vi "MAVLink Driver Main.vi"(8 "error IO":errorcluster) -> ()   [LabVIEW 2014]
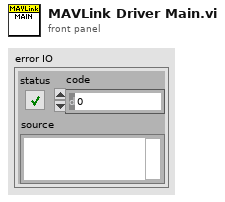
[diagram p1: front panel]
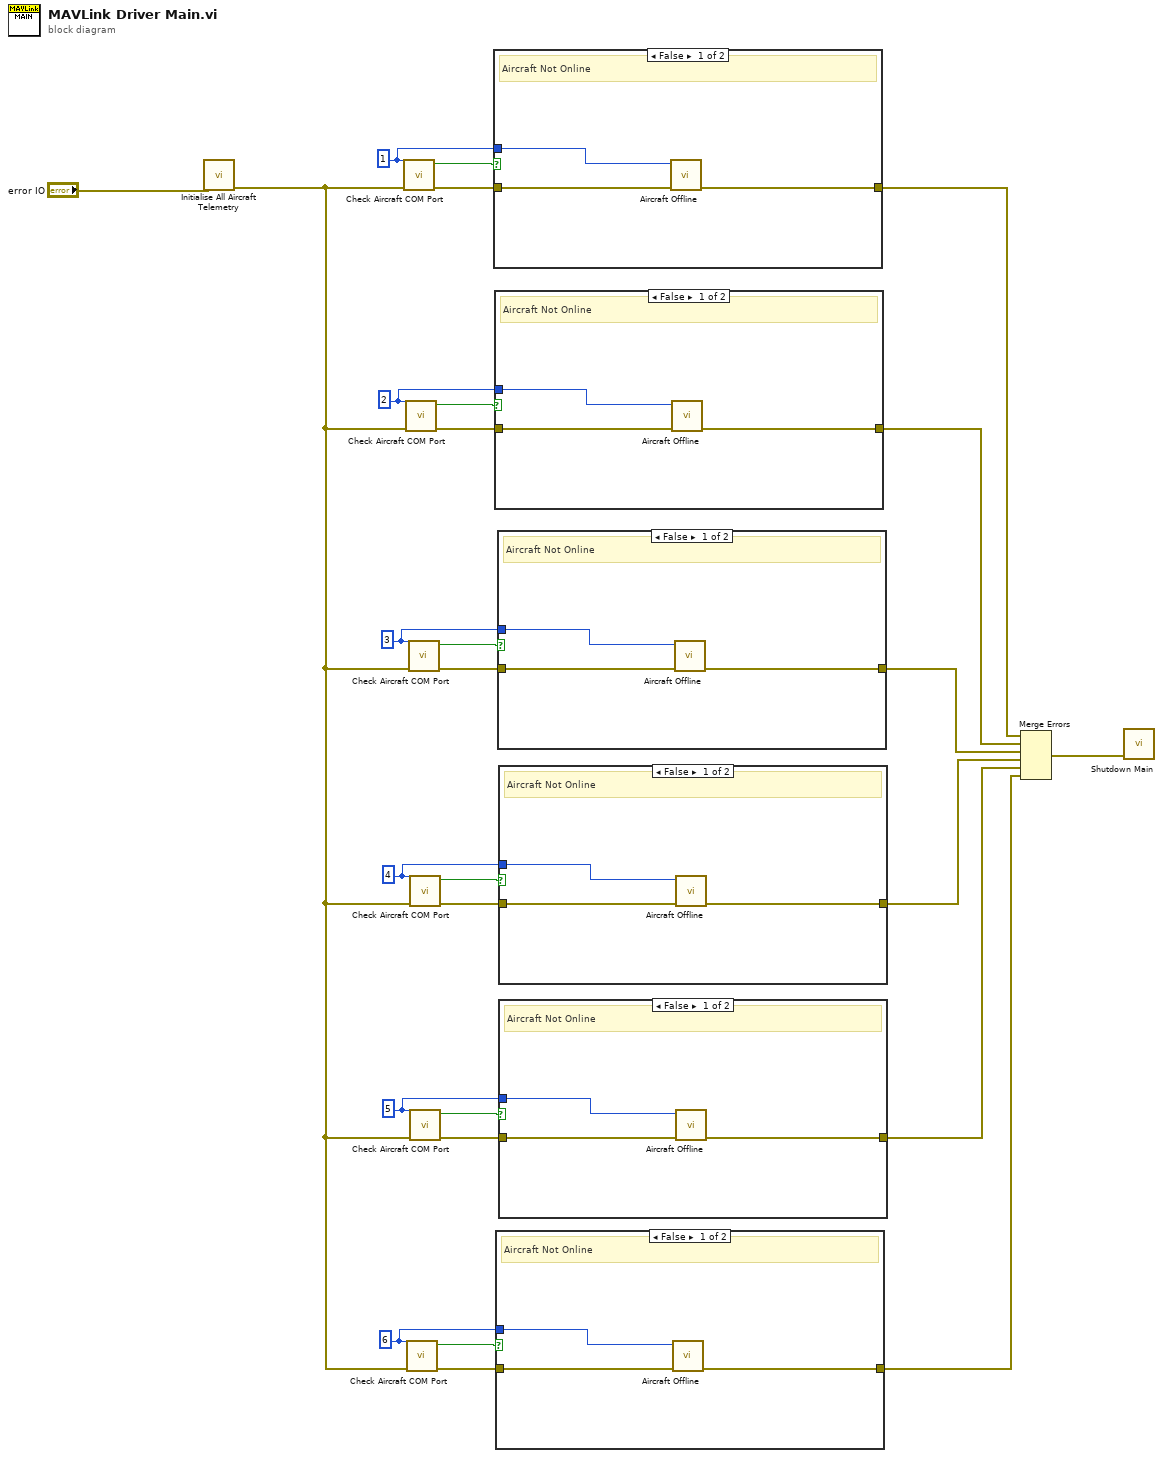
[diagram p0: block diagram]
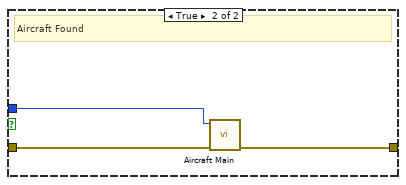
[diagram p2: hidden frame]
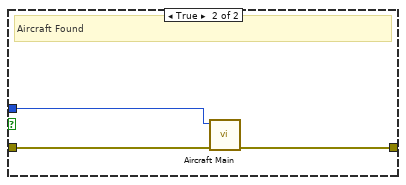
[diagram p3: hidden frame]
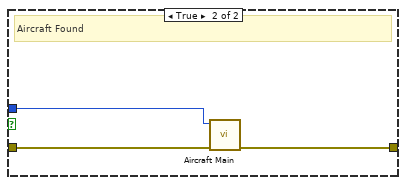
[diagram p4: hidden frame]
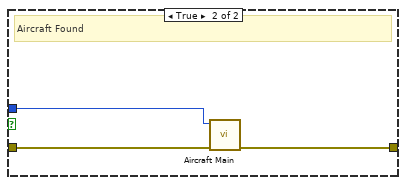
[diagram p5: hidden frame]
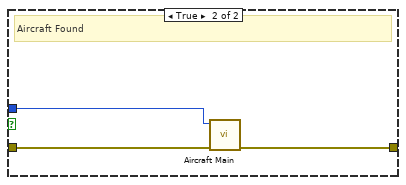
[diagram p6: hidden frame]
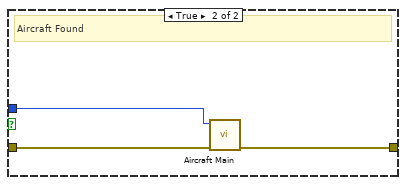
[diagram p7: hidden frame]
diagram:
  w11 = u8 6 ("Aircraft ID")
  w12 = u8 5 ("Aircraft ID")
  w17 = u8 4 ("Aircraft ID")
  w18 = u8 3 ("Aircraft ID")
  w23 = u8 2 ("Aircraft ID")
  w24 = u8 1 ("Aircraft ID")
  n1 = call "Initialise All Aircraft Telemetry.vi"("error IO"="error IO") -> ("error out"=w8:errorcluster)  [unwired: 10 in]
  n2 = call "Check Aircraft COM Port.vi"("Error In"=w8, "Aircraft ID"=w24) -> ("Error Out"=w25:errorcluster, "COM Port Found"=w26:bool)  [unwired: 8 in]
  n3 = call "Check Aircraft COM Port.vi"("Error In"=w8, "Aircraft ID"=w23) -> ("Error Out"=w22:errorcluster, "COM Port Found"=w21:bool)  [unwired: 8 in]
  n4 = call "Check Aircraft COM Port.vi"("Error In"=w8, "Aircraft ID"=w11) -> ("Error Out"=w10:errorcluster, "COM Port Found"=w9:bool)  [unwired: 8 in]
  n5 = call "Check Aircraft COM Port.vi"("Error In"=w8, "Aircraft ID"=w18) -> ("Error Out"=w19:errorcluster, "COM Port Found"=w20:bool)  [unwired: 8 in]
  n6 = call "Check Aircraft COM Port.vi"("Error In"=w8, "Aircraft ID"=w17) -> ("Error Out"=w16:errorcluster, "COM Port Found"=w15:bool)  [unwired: 8 in]
  n7 = call "Check Aircraft COM Port.vi"("Error In"=w8, "Aircraft ID"=w12) -> ("Error Out"=w13:errorcluster, "COM Port Found"=w14:bool)  [unwired: 8 in]
  n8 = case shown="False" w26 {
    tunnel: w25 -> [w29 w33]
    tunnel: w24 -> [w30 w32]
    tunnel: [w28 w31] -> w7
    frame False {
      # "Aircraft Not Online"
      n9 = call "Aircraft Offline.vi"("Error In"=w29, "Aircraft ID"=w30) -> ("Error Out"=w28:errorcluster)  [unwired: 9 in]
    }
    frame True {
      # "Aircraft Found"
      n10 = call "Aircraft Main.vi"("error out"=w33, "Aircraft Index"=w32) -> ("error out 2"=w31:errorcluster)  [unwired: 9 in]
    }
  }
  n11 = case shown="False" w21 {
    tunnel: w22 -> [w35 w39]
    tunnel: w23 -> [w36 w38]
    tunnel: [w34 w37] -> w6
    frame False {
      # "Aircraft Not Online"
      n12 = call "Aircraft Offline.vi"("Error In"=w35, "Aircraft ID"=w36) -> ("Error Out"=w34:errorcluster)  [unwired: 9 in]
    }
    frame True {
      # "Aircraft Found"
      n13 = call "Aircraft Main.vi"("error out"=w39, "Aircraft Index"=w38) -> ("error out 2"=w37:errorcluster)  [unwired: 9 in]
    }
  }
  n14 = case shown="False" w9 {
    tunnel: w10 -> [w41 w45]
    tunnel: w11 -> [w42 w44]
    tunnel: [w40 w43] -> w2
    frame False {
      # "Aircraft Not Online"
      n15 = call "Aircraft Offline.vi"("Error In"=w41, "Aircraft ID"=w42) -> ("Error Out"=w40:errorcluster)  [unwired: 9 in]
    }
    frame True {
      # "Aircraft Found"
      n16 = call "Aircraft Main.vi"("error out"=w45, "Aircraft Index"=w44) -> ("error out 2"=w43:errorcluster)  [unwired: 9 in]
    }
  }
  n17 = case shown="False" w20 {
    tunnel: w19 -> [w47 w51]
    tunnel: w18 -> [w48 w50]
    tunnel: [w46 w49] -> w5
    frame False {
      # "Aircraft Not Online"
      n18 = call "Aircraft Offline.vi"("Error In"=w47, "Aircraft ID"=w48) -> ("Error Out"=w46:errorcluster)  [unwired: 9 in]
    }
    frame True {
      # "Aircraft Found"
      n19 = call "Aircraft Main.vi"("error out"=w51, "Aircraft Index"=w50) -> ("error out 2"=w49:errorcluster)  [unwired: 9 in]
    }
  }
  n20 = case shown="False" w15 {
    tunnel: w16 -> [w53 w57]
    tunnel: w17 -> [w54 w56]
    tunnel: [w52 w55] -> w4
    frame False {
      # "Aircraft Not Online"
      n21 = call "Aircraft Offline.vi"("Error In"=w53, "Aircraft ID"=w54) -> ("Error Out"=w52:errorcluster)  [unwired: 9 in]
    }
    frame True {
      # "Aircraft Found"
      n22 = call "Aircraft Main.vi"("error out"=w57, "Aircraft Index"=w56) -> ("error out 2"=w55:errorcluster)  [unwired: 9 in]
    }
  }
  n23 = case shown="False" w14 {
    tunnel: w13 -> [w59 w63]
    tunnel: w12 -> [w60 w62]
    tunnel: [w58 w61] -> w3
    frame False {
      # "Aircraft Not Online"
      n24 = call "Aircraft Offline.vi"("Error In"=w59, "Aircraft ID"=w60) -> ("Error Out"=w58:errorcluster)  [unwired: 9 in]
    }
    frame True {
      # "Aircraft Found"
      n25 = call "Aircraft Main.vi"("error out"=w63, "Aircraft Index"=w62) -> ("error out 2"=w61:errorcluster)  [unwired: 9 in]
    }
  }
  n26 = Merge Errors(w7, w6, w5, w4, w3, w2) -> (w1:errorcluster)
  n27 = call "Shutdown Main.vi"("error out"=w1) -> ()  [unwired: 11 in]
